vi "pco.labview_Simple_CamRam_Example.vi"() -> ()   [LabVIEW 2019]
uses:
  pco.sdk/CameraAccess/CameraAccess.lvlib
  pco.sdk/Structures/Structures.lvlib
  pco.recorder/Recorder.lvlib
  pco.sdk/RecordingControl/RecordingControl.lvlib
  pco.sdk/TimingControl/TimingControl.lvlib
  pco.sdk/GeneralCameraControl/GeneralCameraControl.lvlib
panel:
  in  "Stop Record":bool
  out "Recording On":bool
  in  "wSegment":u16=1 caption="Ram Segment" min=1 max=4 step=1
  out "Recorded Images":u32
  out "Image":u16[][](graph)
  in  "Quit":bool
  in  "roiY1":u16=2 min=2 step=1
  in  "roiX1":u16=2 min=2 step=1
  in  "roiY0":u16=1 min=1 step=1
  in  "roiX0":u16=1 min=1 step=1
  out "Image Height":u16
  out "Image Width":u16
  in  "Image Index":u32 max=265
  out "Error":errorcluster {"code" format="%x"}
  # "This example shows a simple recording of an image sequence and the image access afterwards for cameras with internal memory.\nIt is a good starting point for writing own applications.\nBut it will not be fail save, i.e. doesnt react on errors, just handles them forward to the end\n\nUsage:\nSelect your required ram segment you start the program.\nOnce started, the camera will be opened and switched to ringbuffer mode.\nThe recorder will be created, initialized and images will be recorded automatically.\nTo stop the recording press the stop record button\nWhen acquisition has finished you can address the images and set a certain roi \nTo finish the program click on quit application, this will force free and delete of the recorder and a close camera"
  # "pco.labview"
  # "Camera Setup"
  # "Recording Control"
  # "Parameters for image readout"
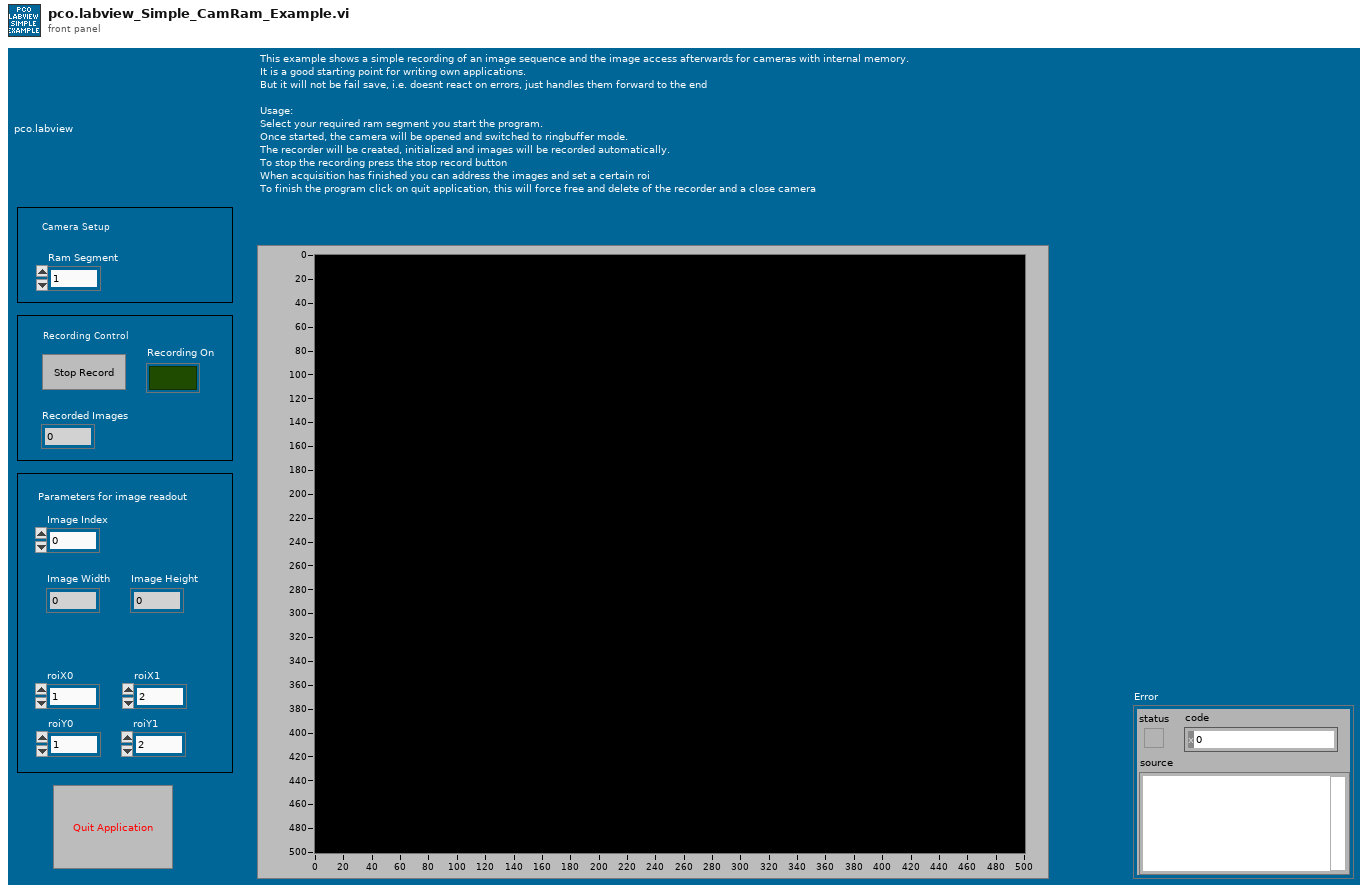
[diagram p1: front panel]
types:
  T1 = enum8{"Enabled", "Disabled", "Disabled and Grayed Out"}
  T2 = cluster{"wInterfaceType":u16, "wCameraNumber":u16, "wCameraNumAtInterface":u16, "wOpenFlags":u16[], "dwOpenFlags":u32[], "wOpenPtr":u64[]}
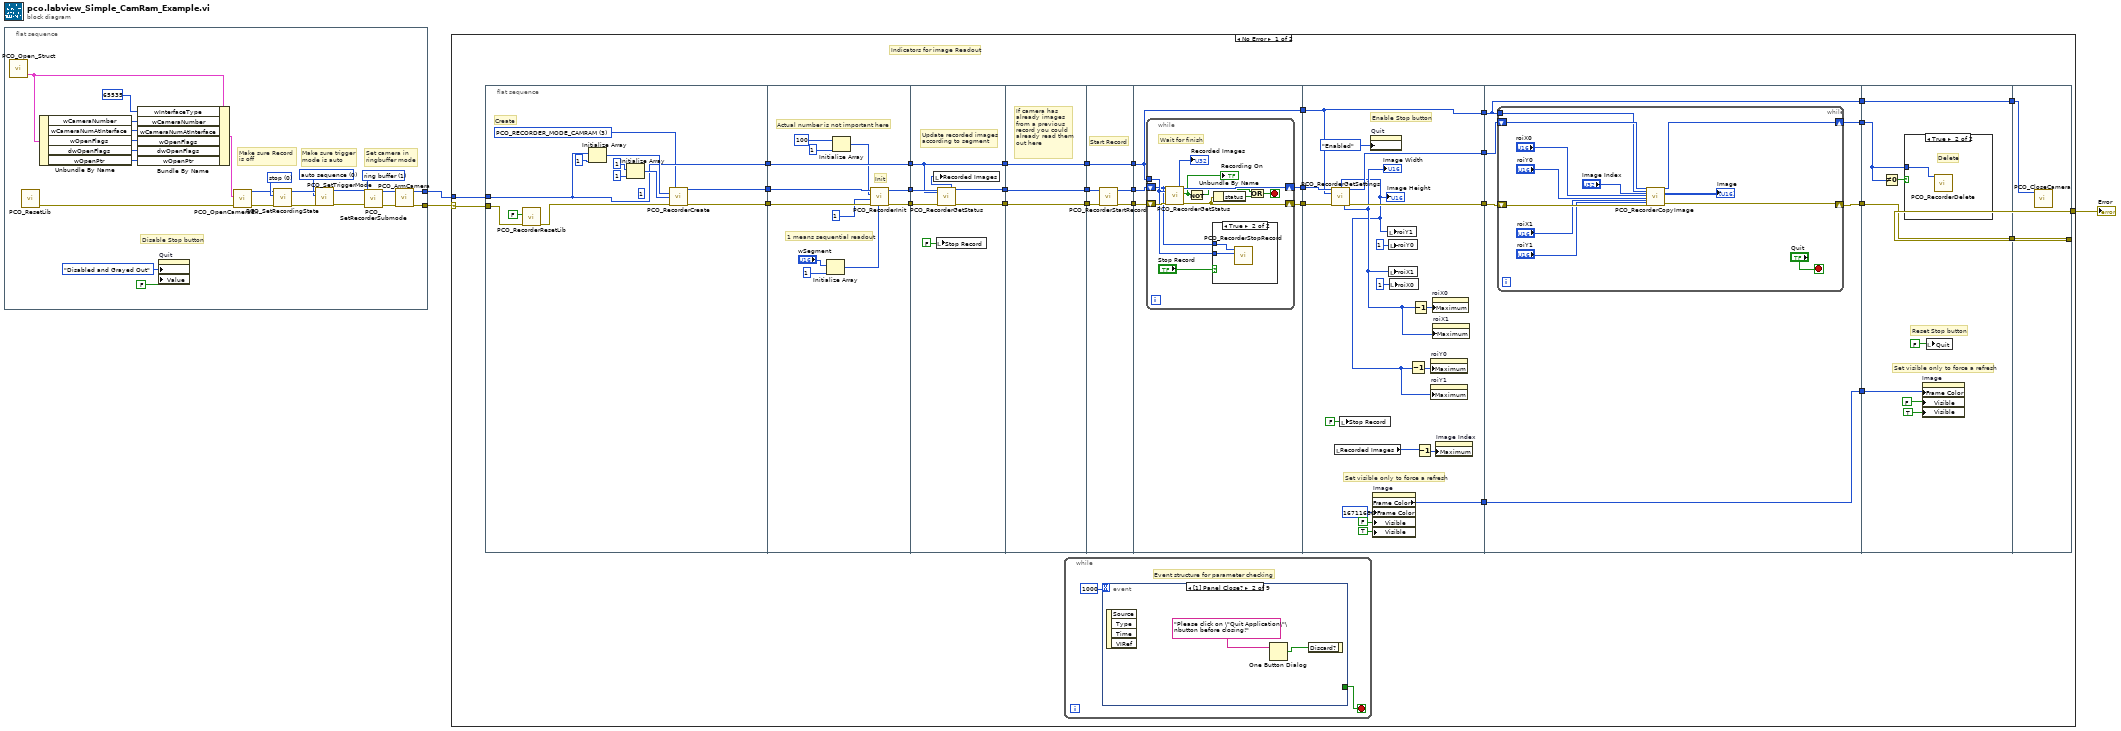
[diagram p0: block diagram]
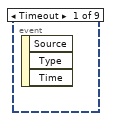
[diagram p2: hidden frame]
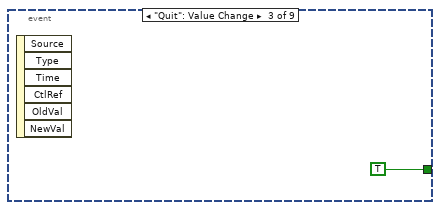
[diagram p3: hidden frame]
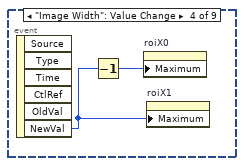
[diagram p4: hidden frame]
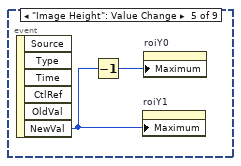
[diagram p5: hidden frame]
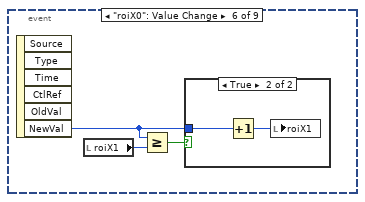
[diagram p6: hidden frame]
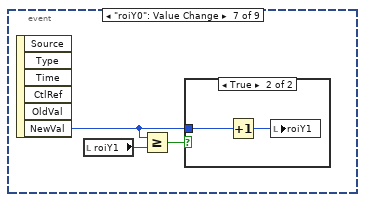
[diagram p8: hidden frame]
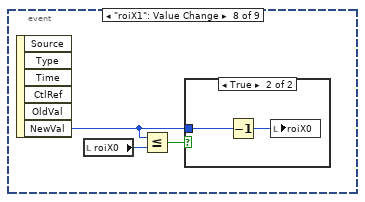
[diagram p10: hidden frame]
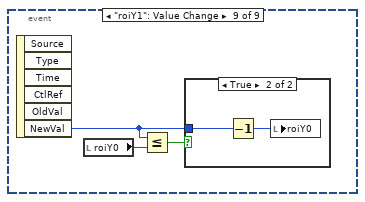
[diagram p12: hidden frame]
diagram:
  n1 = flat-sequence {
    tunnel: [w5] -> w3
    tunnel: [w4] -> w1
    frame #0 {
      w8 = u16 1 items=["sequence", "ring buffer"] ("wRecSubmode")
      w11 = u16 0 items=["auto sequence"=0, "software trigger"=1, "external exposure start & software trigger"=2, "external exposure control"=3, "external synchronized"=4, "fast external exposure control"=5, "external CDS control"=6, "slow external exposure control"=7, "external synchronized HDSDI"=258] ("wTriggerMode")
      w16 = u16 0 items=["stop", "run"] ("wRecState")
      # "Set camera in\nringbuffer mode"
      # "Make sure trigger\nmode is auto"
      # "Make sure Record \nis off"
      # "Disable Stop button"
      n2 = call "PCO_Open_Struct.vi"() -> ("PCO_Open_Struct"=w23:T2)  [unwired: 4 in, 4 out]
      n3 = call "PCO_ResetLib.vi"() -> ("error out"=w27:errorcluster)  [unwired: 10 in, 1 out]
      n4 = Unbundle By Name(w23) -> ("wCameraNumber"=w22:u16, "wCameraNumAtInterface"=w21:u16, "wOpenFlags"=w20:u16[], "dwOpenFlags"=w19:u32[], "wOpenPtr"=w18:u64[])
      n5 = Bundle By Name(cluster=w23, "wInterfaceType"=u16 65535, "wCameraNumber"=w22, "wCameraNumAtInterface"=w21, "wOpenFlags"=w20, "dwOpenFlags"=w19, "wOpenPtr"=w18) -> (w17:T2)
      n6 = property on="Quit" class="Bool (strict)"("DisabledEnum"=T1."Disabled and Grayed Out" ("Disabled"), "Value"=FALSE ("Stop")) -> ()  [unwired: 2 in, 2 out]
      n7 = call "PCO_OpenCameraEx.vi"("error in (no error)"=w27, "strOpenStruct"=w17) -> ("error out"=w15:errorcluster, "ph out"=w14:u64)  [unwired: 7 in, 1 out]
      n8 = call "PCO_SetRecordingState.vi"("error in (no error)"=w15, "wRecState"=w16, "ph"=w14) -> ("error out"=w12:errorcluster, "ph out"=w13:u64)  [unwired: 6 in, 1 out]
      n9 = call "PCO_SetTriggerMode.vi"("error in (no error)"=w12, "wTriggerMode"=w11, "ph"=w13) -> ("error out"=w10:errorcluster, "ph out"=w9:u64)  [unwired: 6 in, 1 out]
      n10 = call "PCO_SetRecorderSubmode.vi"("error in (no error)"=w10, "wRecSubmode"=w8, "ph"=w9) -> ("error out"=w7:errorcluster, "ph out"=w6:u64)  [unwired: 6 in, 1 out]
      n11 = call "PCO_ArmCamera.vi"("error in (no error)"=w7, "ph"=w6) -> ("error out"=w4:errorcluster, "ph out"=w5:u64)  [unwired: 7 in, 1 out]
    }
  }
  n12 = case shown="No Error" w1 {
    selector: w1 -> [w41 w193]
    tunnel: [w37 w193] -> w2
    tunnel: w3 -> [w58 _]
    frame No Error {
      # "Indicators for image Readout"
      n13 = flat-sequence {
        tunnel: w58 -> [w93]
        tunnel: w41 -> [w90]
        tunnel: [w92] -> w57
        tunnel: [w94] -> w56
        tunnel: [w93] -> w48
        tunnel: w57 -> [w111]
        tunnel: w56 -> [w107]
        tunnel: [w110] -> w33
        tunnel: [w109] -> w31
        tunnel: [w108] -> w29
        tunnel: w48 -> [w108]
        tunnel: w33 -> [w117]
        tunnel: [w116] -> w32
        tunnel: w31 -> [w115]
        tunnel: [w114] -> w30
        tunnel: w29 -> [w113]
        tunnel: [w113] -> w28
        tunnel: w32 -> [w121]
        tunnel: [w121] -> w36
        tunnel: w30 -> [w120]
        tunnel: [w120] -> w35
        tunnel: w28 -> [w119]
        tunnel: [w119] -> w34
        tunnel: w36 -> [w126]
        tunnel: w35 -> [w125]
        tunnel: [w124] -> w55
        tunnel: [w123] -> w54
        tunnel: [w122] -> w49
        tunnel: w34 -> [w122]
        tunnel: w55 -> [w131]
        tunnel: w54 -> [w130]
        tunnel: [w129] -> w53
        tunnel: [w128] -> w52
        tunnel: w49 -> [w127]
        tunnel: [w127] -> w47
        tunnel: w53 -> [w162]
        tunnel: w52 -> [w161]
        tunnel: [w160] -> w51
        tunnel: [w159] -> w50
        tunnel: w47 -> [w158]
        tunnel: [w158] -> w46
        tunnel: [w154] -> w40
        tunnel: w51 -> [w169]
        tunnel: w50 -> [w168]
        tunnel: w46 -> [w165]
        tunnel: [w167] -> w45
        tunnel: [w166] -> w44
        tunnel: [w165] -> w43
        tunnel: w40 -> [w164]
        tunnel: [w164] -> w39
        tunnel: w45 -> [w182]
        tunnel: w44 -> [w188]
        tunnel: w43 -> [w186]
        tunnel: [w186] -> w42
        tunnel: w39 -> [w183]
        tunnel: [w182] -> w38
        tunnel: w42 -> [w192]
        tunnel: w38 -> [w191]
        tunnel: [w191] -> w37
        frame #0 {
          w88 = u16 3 items=["PCO_RECORDER_MODE_FILE"=1, "PCO_RECORDER_MODE_MEMORY"=2, "PCO_RECORDER_MODE_CAMRAM"=3] ("dwRecMode")
          (unwired) u16 1 ("wArrLength")
          # "Create"
          n14 = call "PCO_RecorderResetLib.vi"("error in (no error)"=w90, "bSilent"=FALSE) -> ("error out"=w89:errorcluster)  [unwired: 8 in, 1 out]
          n15 = Initialize Array(w93, u32 1 ("element")) -> (w98:u64[])
          n16 = Initialize Array(u32 1 ("element"), u32 1 ("element")) -> (w95:u32[])
          n17 = call "PCO_RecorderCreate.vi"("wRecMode"=w88, "phCamArr"=w98, "dwImgDistributionArr"=w95, "error in (no error)"=w89) -> ("phRec out"=w92:u64, "error out"=w94:errorcluster)  [unwired: 8 in, 2 out]
        }
        frame #1 {
          # "Actual number is not important here"
          # "1 means sequential readout"
          # "Init"
          n18 = Initialize Array("wSegment", 1 ("dimension size")) -> (w101:u16[])
          n19 = Initialize Array(u32 100 ("dimension size"), 1 ("dimension size")) -> (w105:u32[])
          n20 = call "PCO_RecorderInit.vi"("wRamSegmentArr"=w101, "error in (no error)"=w107, "wType"=u16 1, "dwImgCountArr"=w105, "phRec"=w111) -> ("error out"=w109:errorcluster, "phRec out"=w110:u64)  [unwired: 4 in, 1 out]
        }
        frame #2 {
          # "Update recorded images\naccording to segment"
          n21 = local write "Stop Record"(FALSE ("Stop Record")) -> ()
          n22 = call "PCO_RecorderGetStatus.vi"("phRec"=w117, "phCam"=w113, "error in (no error)"=w115) -> ("dwProcImgCount"=w118:u32, "phRec out"=w116:u64, "error out"=w114:errorcluster)  [unwired: 5 in, 9 out]
          n23 = local write "Recorded Images"(w118) -> ()
        }
        frame #3 {
          # "If camera has \nalready images\nfrom a previous\nrecord you could\nalready read them\nout here"
        }
        frame #4 {
          # "Start Record"
          n24 = call "PCO_RecorderStartRecord.vi"("error in (no error)"=w125, "phRec"=w126) -> ("error out"=w124:errorcluster, "phRec out"=w123:u64)  [unwired: 7 in, 1 out]
        }
        frame #5 {
          n25 = while {
            shift-right: [w141] -> w128
            shift-left: w131 -> [w142]
            shift-right: [w138] -> w129
            shift-left: w130 -> [w132]
            tunnel: w127 -> [w133]
            stop <- w139 stop-if-true
            # "Wait for finish"
            n26 = call "PCO_RecorderGetStatus.vi"("phRec"=w132, "phCam"=w133, "error in (no error)"=w142) -> ("dwProcImgCount"=→"Recorded Images":u32, "phRec out"=w138:u64, "bIsRunning"=w135:bool, "error out"=w141:errorcluster)  [unwired: 5 in, 8 out]
            "Recording On" <- w135
            n27 = Not(x=w135) -> (.not. x?=w137:bool)
            n28 = case shown="True" "Stop Record" {
              tunnel: w133 -> [_ w144]
              tunnel: w132 -> [_ w143]
              frame False {
              }
              frame True {
                n29 = call "PCO_RecorderStopRecord.vi"("phCam"=w144, "phRec"=w143) -> ()  [unwired: 7 in, 3 out]
              }
            }
            n30 = Unbundle By Name(w141) -> ("status"=w140:bool)
            n31 = Or(x=w137, y=w140) -> (x .or. y?=w139:bool)
          }
        }
        frame #6 {
          # "Set visible only to force a refresh"
          # "Enable Stop button"
          n32 = call "PCO_RecorderGetSettings.vi"("phRec"=w162, "phCam"=w158, "error in (no error)"=w161) -> ("wHeight"=w147:u16, "phRec out"=w160:u64, "wWidth"=w148:u16, "error out"=w159:errorcluster)  [unwired: 4 in, 5 out]
          "Image Width" <- w148
          "Image Height" <- w147
          n33 = local read "Recorded Images"() -> (w146:u32)
          n34 = local write "Stop Record"(FALSE ("Stop Record")) -> ()
          n35 = property on="Quit" class="Bool (strict)"("DisabledEnum"=T1."Enabled" ("Disabled")) -> ()  [unwired: 2 in, 2 out]
          n36 = property on="Image" class="IntGraph (strict)"("Frame Color"=u32 16711680, "Visible"=FALSE, "Visible"=TRUE) -> ("Frame Color"=w154:u32)  [unwired: 2 in, 2 out]
          n37 = local write "roiY1"(w147) -> ()
          n38 = local write "roiY0"(u16 1 ("roiY0")) -> ()
          n39 = local write "roiX1"(w148) -> ()
          n40 = local write "roiX0"(u16 1 ("roiY0")) -> ()
          n41 = Decrement(x=w147) -> (x-1=w150:u16)
          n42 = Decrement(x=w148) -> (x-1=w151:u16)
          n43 = Decrement(x=w146) -> (x-1=w149:u32)
          n44 = property on="roiY0" class="DigNum (strict)"("Maximum"=w150) -> ()  [unwired: 2 in, 2 out]
          n45 = property on="roiY1" class="DigNum (strict)"("Maximum"=w147) -> ()  [unwired: 2 in, 2 out]
          n46 = property on="roiX0" class="DigNum (strict)"("Maximum"=w151) -> ()  [unwired: 2 in, 2 out]
          n47 = property on="roiX1" class="DigNum (strict)"("Maximum"=w148) -> ()  [unwired: 2 in, 2 out]
          n48 = property on="Image Index" class="DigNum (strict)"("Maximum"=w149) -> ()  [unwired: 2 in, 2 out]
        }
        frame #7 {
          n49 = while {
            tunnel: w165 -> [w178]
            shift-right: [w177] -> w166
            shift-left: w169 -> [w180]
            shift-right: [w176] -> w167
            shift-left: w168 -> [w179]
            stop <- "Quit" stop-if-true
            n50 = call "PCO_RecorderCopyImage.vi"("phRec"=w180, "phCam"=w178, "dwImgIdx"="Image Index", "wRoiX0"="roiX0", "wRoiY0"="roiY0", "wRoiX1"="roiX1", "wRoiY1"="roiY1", "error in (no error)"=w179) -> ("phRec out"=w177:u64, "wImgBuf"=→"Image":u16[][], "error out"=w176:errorcluster)  [unwired: 13 in, 4 out]
          }
        }
        frame #8 {
          # "Set visible only to force a refresh"
          # "Reset Stop button"
          n51 = Not Equal To 0?(x=w188) -> (x != 0?=w187:bool)
          n52 = case shown="True" w187 {
            tunnel: w188 -> [_ w190]
            frame False {
            }
            frame True {
              # "Delete"
              n53 = call "PCO_RecorderDelete.vi"("phRec"=w190) -> ()  [unwired: 9 in, 2 out]
            }
          }
          n54 = property on="Image" class="IntGraph (strict)"("Frame Color"=w183, "Visible"=FALSE, "Visible"=TRUE) -> ()  [unwired: 2 in, 2 out]
          n55 = local write "Quit"(FALSE ("Stop")) -> ()
        }
        frame #9 {
          n56 = call "PCO_CloseCamera.vi"("ph"=w192) -> ()  [unwired: 9 in, 2 out]
        }
      }
      n57 = while {
        stop <- w59 stop-if-true
        # "Event structure for parameter checking"
        n58 = event shown="[1] Panel Close?" {
          selector: _ -> [_ _ _ _ _ _ _ _ _]
          dyn-events: _ -> [_ _ _ _ _ _ _ _ _]
          timeout: 1000 -> [_ _ _ _ _ _ _ _ _]
          tunnel: [_ _ TRUE _ _ _ _ _ _] -> w59
          event Timeout {
            n59 = event-data() -> ()  [unwired: 1 in, 3 out]
          }
          event Panel Close? {
            n60 = event-data() -> ()  [unwired: 1 in, 4 out]
            n61 = One Button Dialog(message="Please click on \"Quit Application\"\nbutton before closing!") -> (true=w61:bool)  [unwired: 1 in]
            n62 = event-data("Discard?"=w61) -> ()  [unwired: 1 in, 1 out]
          }
          event "Quit": Value Change {
            n63 = event-data() -> ()  [unwired: 1 in, 6 out]
          }
          event "Image Width": Value Change {
            n64 = event-data() -> ("NewVal"=w64:u16)  [unwired: 1 in, 5 out]
            n65 = Decrement(x=w64) -> (x-1=w65:u16)
            n66 = property on="roiX0" class="DigNum (strict)"("Maximum"=w65) -> ()  [unwired: 2 in, 2 out]
            n67 = property on="roiX1" class="DigNum (strict)"("Maximum"=w64) -> ()  [unwired: 2 in, 2 out]
          }
          event "Image Height": Value Change {
            n68 = event-data() -> ("NewVal"=w66:u16)  [unwired: 1 in, 5 out]
            n69 = Decrement(x=w66) -> (x-1=w67:u16)
            n70 = property on="roiY1" class="DigNum (strict)"("Maximum"=w66) -> ()  [unwired: 2 in, 2 out]
            n71 = property on="roiY0" class="DigNum (strict)"("Maximum"=w67) -> ()  [unwired: 2 in, 2 out]
          }
          event "roiX0": Value Change {
            n72 = event-data() -> ("NewVal"=w68:u16)  [unwired: 1 in, 5 out]
            n73 = local read "roiX1"() -> (w70:u16)
            n74 = Greater Or Equal?(x=w68, y=w70) -> (x >= y?=w69:bool)
            n75 = case shown="True" w69 {
              tunnel: w68 -> [_ w72]
              frame False {
              }
              frame True {
                n76 = Increment(x=w72) -> (x+1=w71:u16)
                n77 = local write "roiX1"(w71) -> ()
              }
            }
          }
          event "roiY0": Value Change {
            n78 = event-data() -> ("NewVal"=w73:u16)  [unwired: 1 in, 5 out]
            n79 = local read "roiY1"() -> (w75:u16)
            n80 = Greater Or Equal?(x=w73, y=w75) -> (x >= y?=w74:bool)
            n81 = case shown="True" w74 {
              tunnel: w73 -> [_ w77]
              frame False {
              }
              frame True {
                n82 = Increment(x=w77) -> (x+1=w76:u16)
                n83 = local write "roiY1"(w76) -> ()
              }
            }
          }
          event "roiX1": Value Change {
            n84 = event-data() -> ("NewVal"=w78:u16)  [unwired: 1 in, 5 out]
            n85 = local read "roiX0"() -> (w80:u16)
            n86 = Less Or Equal?(x=w78, y=w80) -> (x <= y?=w79:bool)
            n87 = case shown="True" w79 {
              tunnel: w78 -> [_ w82]
              frame False {
              }
              frame True {
                n88 = Decrement(x=w82) -> (x-1=w81:u16)
                n89 = local write "roiX0"(w81) -> ()
              }
            }
          }
          event "roiY1": Value Change {
            n90 = event-data() -> ("NewVal"=w83:u16)  [unwired: 1 in, 5 out]
            n91 = local read "roiY0"() -> (w85:u16)
            n92 = Less Or Equal?(x=w83, y=w85) -> (x <= y?=w84:bool)
            n93 = case shown="True" w84 {
              tunnel: w83 -> [_ w87]
              frame False {
              }
              frame True {
                n94 = Decrement(x=w87) -> (x-1=w86:u16)
                n95 = local write "roiY0"(w86) -> ()
              }
            }
          }
        }
      }
    }
    frame Error {
    }
  }
  "Error" <- w2
